vi "CAMERA_main.vi"(1 "Camera type":string) -> ()   [LabVIEW 2015]
uses:
  GLOBAL/Global_CAMERA_TYPE.vi
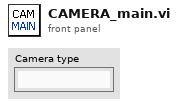
[diagram p1: front panel]
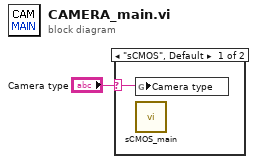
[diagram p0: block diagram]
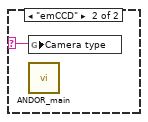
[diagram p2: hidden frame]
diagram:
  n1 = case shown="\"sCMOS\", Default" "Camera type" {
    selector: "Camera type" -> [w2 w3]
    frame "sCMOS", Default {
      n2 = global write "Global_CAMERA_TYPE.vi" "Camera type"(w2) -> ()
      n3 = call "sCMOS_main.vi"() -> ()  [unwired: 12 in]
    }
    frame "emCCD" {
      n4 = global write "Global_CAMERA_TYPE.vi" "Camera type"(w3) -> ()
      n5 = call "ANDOR_main.vi"() -> ()  [unwired: 12 in]
    }
  }
